vi "TPNT_PeriodicUpdate.vi"(4 "deflogsep":string="blank", 5 "UTC":bool, 6 "notifier":refnum<notifier>, 7 "mailserver":string="localhost", 9 "log":bool, 10 "logfile":path, 11 "queueIn":refnum<queue>) -> ()   [LabVIEW 2016]
uses:
  TPNT_CoreFunction.ctl
  TPNT_Refnum.ctl
panel:
  in  "sample now":bool
  in  "pause":bool
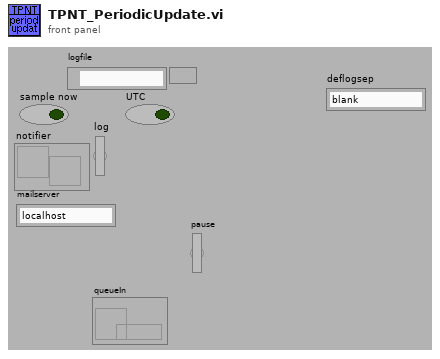
[diagram p1: front panel]
types:
  T1 = typedef "TPNT_Refnum.ctl" = refnum<vi>
  T2 = typedef "TPNT_CoreFunction.ctl" = enum16{"Reset", "Register", "Get Data", "Set Data", "Unregister", "Test", "Get Objects"}
  T3 = typedef "TPNT_TP.ctl" = cluster{"name":string, "type":string, "algor":string[], "update_rate":sgl, "Limits":T4, "Samples":T5, "next_update":u32, "Status":string, "monitor":bool, "error":bool, "Log":T6, "permissions":string, "ID":string}
  T4 = typedef "TPNT_Limits.ctl" = cluster{"Alarm Type":string, "Lower ":dbl, "Upper":dbl, "Nominal":dbl, "outrange":bool, "Check":bool, "latch":bool, "level":string}
  T5 = typedef "TPNT_Samples.ctl" = cluster{"samples":i32, "counter":i32, "Values":dbl[], "Current Value":string, "filter":string, "precision":u8}
  T6 = typedef "TPNT_Log.ctl" = cluster{"log":bool, "file":path, "type":string, "format":string, "updaterate":dbl, "nex_update":u32, "mode":string}
  T7 = typedef "TPNT_DeviceTPs.ctl" = cluster{"device":string, "devupdate":dbl, "next_update":u32, "devinterface":string, "TPs":T3[], "Alarms":bool, "monitor":bool, "log sep":string}
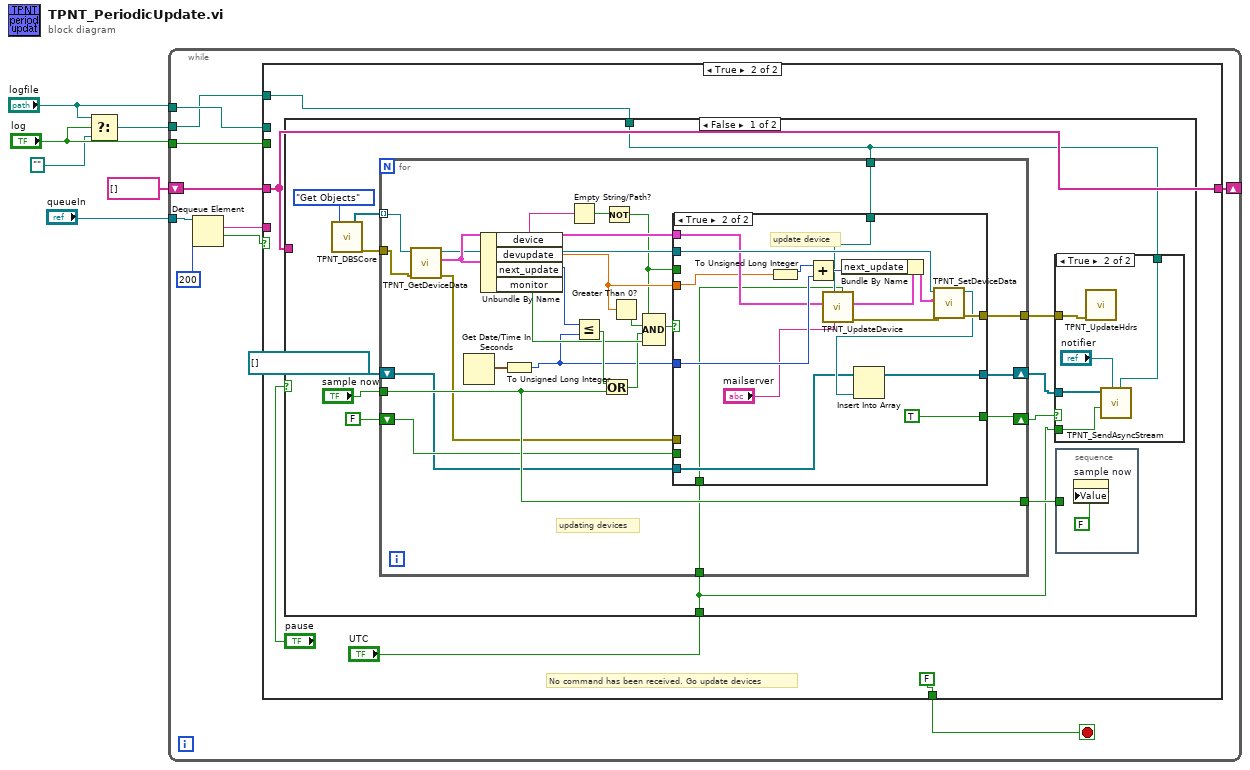
[diagram p0: block diagram]
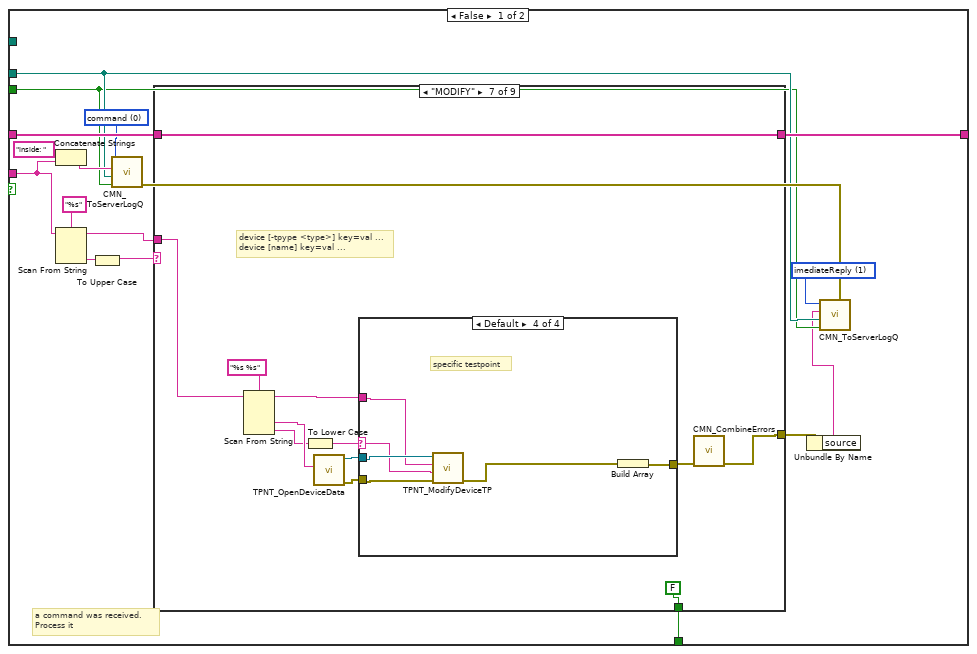
[diagram p2: hidden frame]
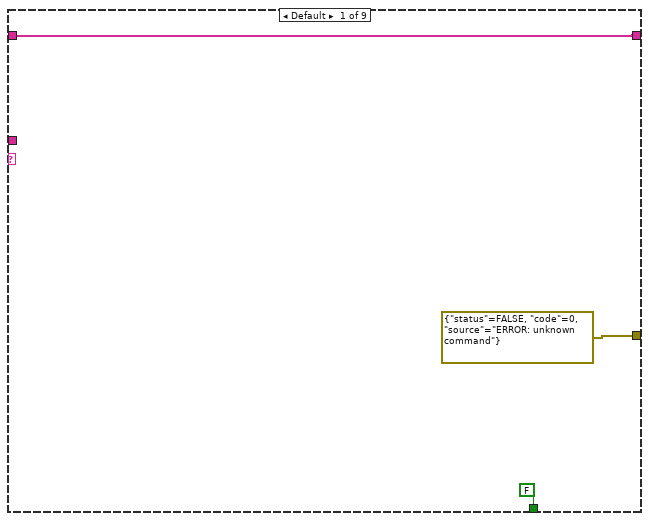
[diagram p3: hidden frame]
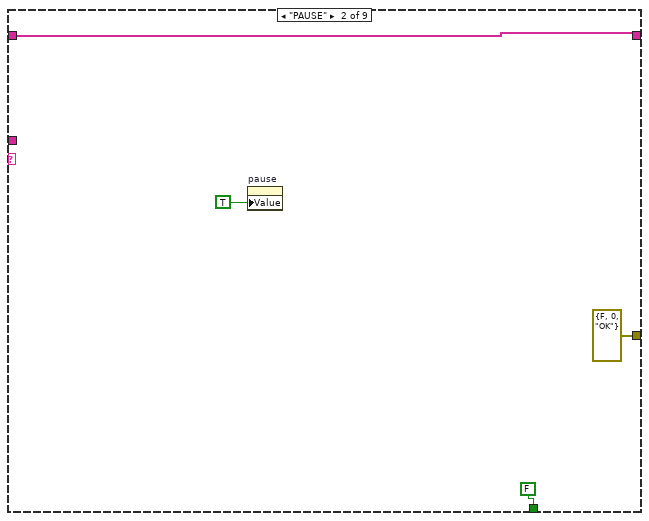
[diagram p4: hidden frame]
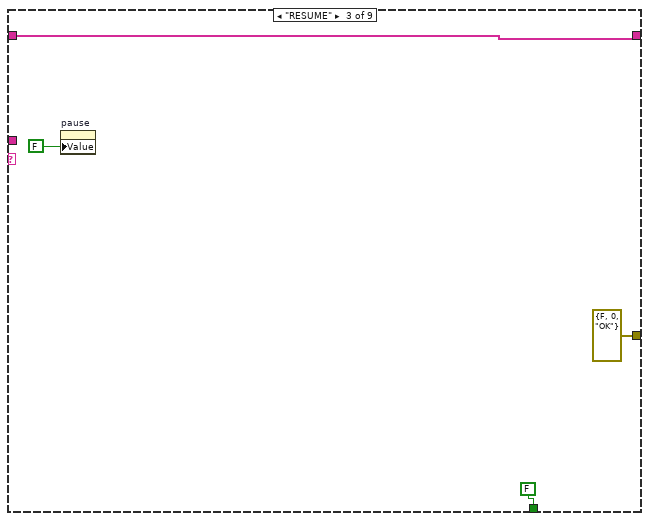
[diagram p5: hidden frame]
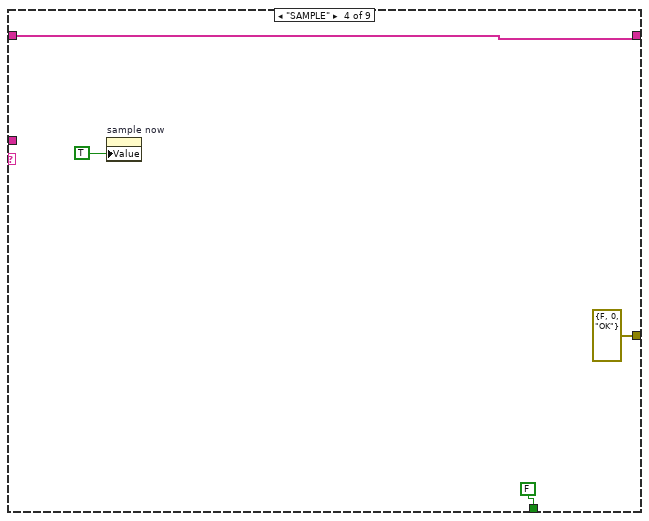
[diagram p6: hidden frame]
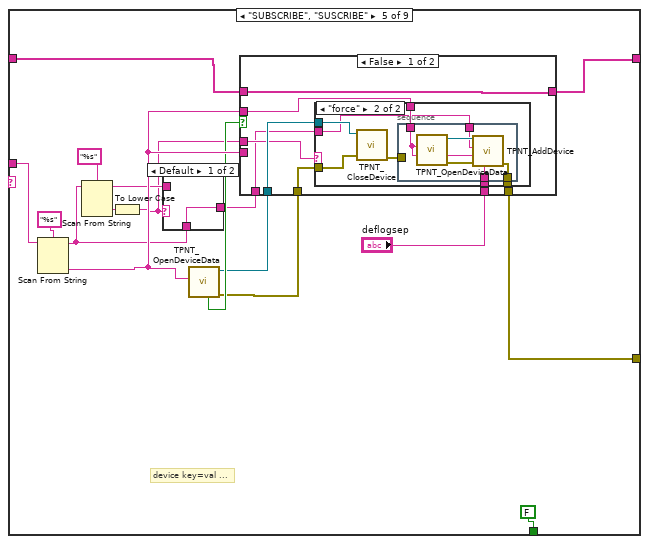
[diagram p7: hidden frame]
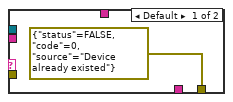
[diagram p9: hidden frame]
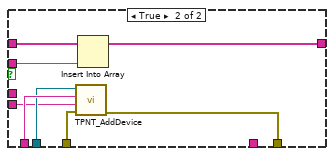
[diagram p10: hidden frame]
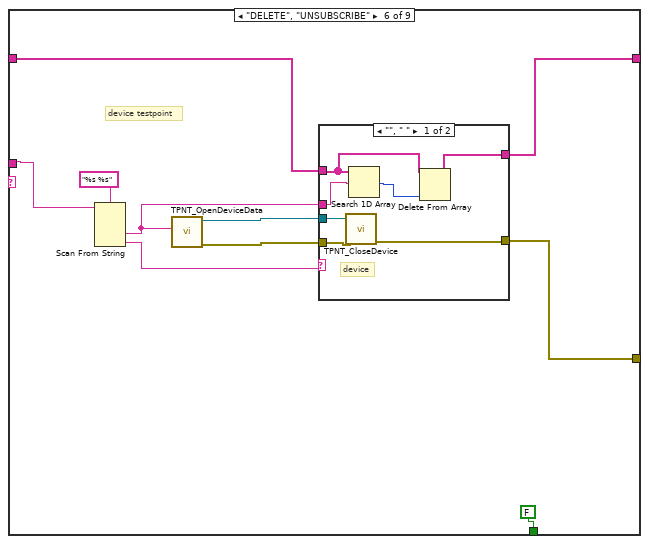
[diagram p11: hidden frame]
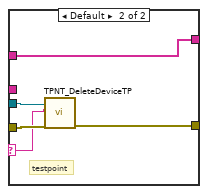
[diagram p12: hidden frame]
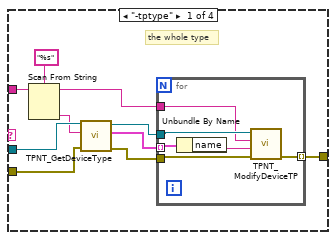
[diagram p13: hidden frame]
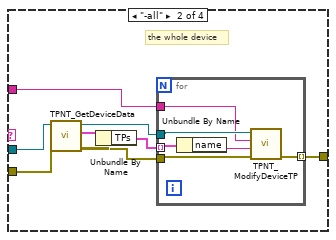
[diagram p14: hidden frame]
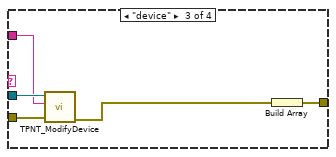
[diagram p15: hidden frame]
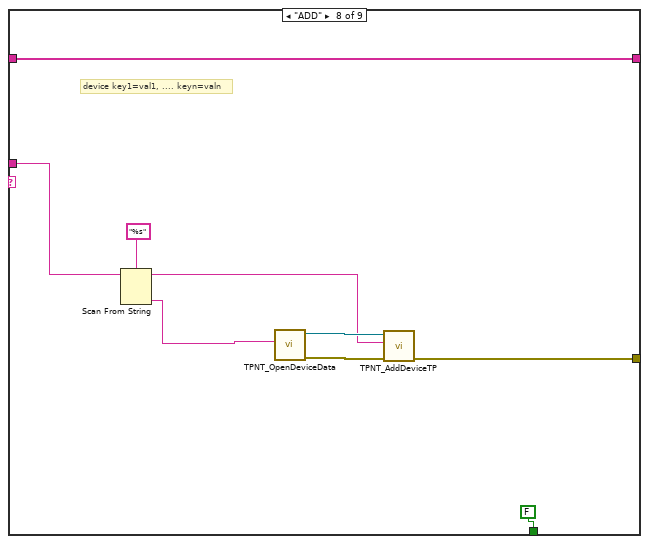
[diagram p16: hidden frame]
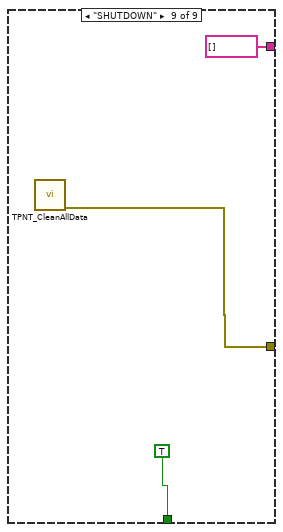
[diagram p17: hidden frame]
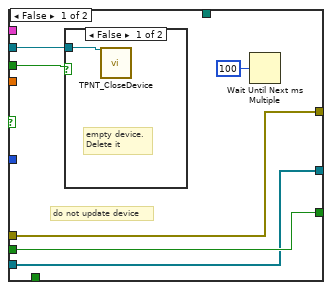
[diagram p19: hidden frame]
diagram:
  n1 = Select(t="logfile", s="log", f=path "") -> (s? t:f=w1:path)
  n2 = while {
    tunnel: "queueIn" -> [w16]
    shift-right: [w12] -> _
    shift-left: string[] [] -> [w10]
    tunnel: "log" -> [w9]
    tunnel: "logfile" -> [w8]
    tunnel: w1 -> [w7]
    stop <- w11 stop-if-true
    n3 = Dequeue Element(queue=w16, timeout in ms (-1)=200) -> (element=w13:string, timed out?=w14:bool)  [unwired: 1 in, 2 out]
    n4 = case shown="True" w14 {
      tunnel: w10 -> [w29 w188]
      tunnel: w13 -> [w24 _]
      tunnel: [w28 w188] -> w12
      tunnel: [w27 FALSE] -> w11
      tunnel: w9 -> [w20 _]
      tunnel: w8 -> [w21 _]
      tunnel: w7 -> [_ w186]
      frame False {
        w19 = u16 1 items=["command", "imediateReply", "Callback Reply", "Information"] ("type")
        w26 = u16 0 items=["command", "imediateReply", "Callback Reply", "Information"] ("type")
        # "a command was received.\nProcess it"
        n5 = Concatenate Strings("inside: " ("string"), w24) -> (w23:string)
        n6 = Scan From String(format string="%s", input string=w24) -> (remaining string=w30:string, output 1=w33:string)  [unwired: 2 in, 3 out]
        n7 = To Upper Case(1:w33) -> (0:w31:string)
        n8 = call "CMN_ToServerLogQ.vi"("Log"=w20, "file"=w21, "string"=w23, "type"=w26) -> ("error out"=w22:errorcluster)  [unwired: 2 in, 4 out]
        n9 = case shown="\"MODIFY\"" w31 {
          tunnel: w30 -> [_ _ _ _ w64 w101 w124 w177 _]
          tunnel: w29 -> [w35 w39 w43 w48 w63 w99 w122 w175 _]
          tunnel: [w35 w39 w43 w48 w62 w100 w122 w175 string[] []] -> w28
          tunnel: [FALSE FALSE FALSE FALSE FALSE FALSE FALSE FALSE TRUE] -> w27
          tunnel: [errorcluster {"status"=FALSE, "code"=0, "source"="ERROR: unknown command"} ("error out") errorcluster {"status"=FALSE, "code"=0, "source"="OK"} ("error out") errorcluster {"status"=FALSE, "code"=0, "source"="OK"} ("error out") errorcluster {"status"=FALSE, "code"=0, "source"="OK"} ("error out") w56 w98 w120 w173 w182] -> w18
          frame Default {
          }
          frame "PAUSE" {
            n10 = property on="pause" class="Bool (strict)"("Value"=TRUE ("pause")) -> ()  [unwired: 2 in, 2 out]
          }
          frame "RESUME" {
            n11 = property on="pause" class="Bool (strict)"("Value"=FALSE ("pause")) -> ()  [unwired: 2 in, 2 out]
          }
          frame "SAMPLE" {
            n12 = property on="sample now" class="Bool (strict)"("Value"=TRUE ("sample now")) -> ()  [unwired: 2 in, 2 out]
          }
          frame "SUBSCRIBE", "SUSCRIBE" {
            # "device key=val ..."
            n13 = Scan From String(format string="%s", input string=w64) -> (remaining string=w52:string, output 1=w60:string)  [unwired: 2 in, 3 out]
            n14 = Scan From String(format string="%s", input string=w52) -> (remaining string=w51:string, output 1=w54:string)  [unwired: 2 in, 3 out]
            n15 = To Lower Case(string=w54) -> (all lower case string=w50:string)
            n16 = case shown="Default" w50 {
              tunnel: w52 -> [w66 _]
              tunnel: [w66 w67] -> w53
              tunnel: w51 -> [_ w67]
              frame Default {
              }
              frame "force" {
              }
            }
            n17 = call "TPNT_OpenDeviceData.vi"("Name"=w60) -> ("error out"=w57:errorcluster, "Data Refnum out"=w58:T1, "Created New"=w59:bool)  [unwired: 1 in, 7 out]
            n18 = case shown="False" w59 {
              tunnel: w63 -> [w75 w97]
              tunnel: [w75 w96] -> w62
              tunnel: w60 -> [w70 w95]
              tunnel: w53 -> [w69 w94]
              tunnel: w58 -> [w74 w93]
              tunnel: w57 -> [w73 w92]
              tunnel: w60 -> [_ w91]
              tunnel: [w72 w90] -> w56
              tunnel: w50 -> [w71 _]
              tunnel: "deflogsep" -> [w68 _]
              frame False {
                n19 = case shown="\"force\"" w71 {
                  tunnel: w74 -> [_ w81]
                  tunnel: w73 -> [_ w83]
                  tunnel: [errorcluster {"status"=FALSE, "code"=0, "source"="Device already existed"} ("error out") w82] -> w72
                  tunnel: w70 -> [_ w80]
                  tunnel: w69 -> [_ w78]
                  tunnel: w68 -> [_ w77]
                  frame Default {
                  }
                  frame "force" {
                    n20 = call "TPNT_CloseDevice.vi"("error in (no error)"=w83, "Object Refnum In"=w81) -> ("error out"=w79:errorcluster)  [unwired: 9 out]
                    n21 = stacked-sequence {
                      tunnel: [w89] -> w82
                      tunnel: w80 -> [w86]
                      tunnel: w79 -> [_]
                      tunnel: w78 -> [w85]
                      tunnel: w77 -> [w84]
                      frame #0 {
                        n22 = call "TPNT_OpenDeviceData.vi"("Name"=w86) -> ("error out"=w88:errorcluster, "Data Refnum out"=w87:T1)  [unwired: 1 in, 8 out]
                        n23 = call "TPNT_AddDevice.vi"("deflogsep"=w84, "error in (no error)"=w88, "name"=w86, "arguments"=w85, "Object Refnum In"=w87) -> ("error out"=w89:errorcluster)  [unwired: 6 out]
                      }
                    }
                  }
                }
              }
              frame True {
                n24 = call "TPNT_AddDevice.vi"("error in (no error)"=w92, "name"=w91, "arguments"=w94, "Object Refnum In"=w93) -> ("error out"=w90:errorcluster)  [unwired: 1 in, 6 out]
                n25 = Insert Into Array(array=w97, new element=w95) -> (w96:string[])  [unwired: 1 in]
              }
            }
          }
          frame "DELETE", "UNSUBSCRIBE" {
            # "device testpoint"
            n26 = Scan From String(format string="%s %s", input string=w101) -> (output 1=w102:string, output 2=w103:string)  [unwired: 2 in, 5 out]
            n27 = call "TPNT_OpenDeviceData.vi"("Name"=w102) -> ("error out"=w104:errorcluster, "Data Refnum out"=w105:T1)  [unwired: 1 in, 8 out]
            n28 = case shown="\"\", \" \"" w103 {
              selector: w103 -> [_ w117]
              tunnel: w105 -> [w113 w119]
              tunnel: w104 -> [w114 w118]
              tunnel: w102 -> [w109 _]
              tunnel: w99 -> [w110 w116]
              tunnel: [w111 w116] -> w100
              tunnel: [w108 w115] -> w98
              frame "", " " {
                # "device"
                n29 = call "TPNT_CloseDevice.vi"("error in (no error)"=w114, "Object Refnum In"=w113) -> ("error out"=w108:errorcluster)  [unwired: 9 out]
                n30 = Search 1D Array(1D array=w110, element=w109) -> (index of element=w112:i32)  [unwired: 1 out]
                n31 = Delete From Array(array=w110, index=w112) -> (array with subset deleted=w111:string[])  [unwired: 1 in, 1 out]
              }
              frame Default {
                # "testpoint"
                n32 = call "TPNT_DeleteDeviceTP.vi"("error in (no error)"=w118, "TP name"=w117, "Object Refnum In"=w119) -> ("error out"=w115:errorcluster)  [unwired: 8 out]
              }
            }
          }
          frame "MODIFY" {
            # "device [-tpype <type>] key=val ...\ndevice [name] key=val ..."
            n33 = Scan From String(format string="%s %s", input string=w124) -> (remaining string=w127:string, output 1=w130:string, output 2=w126:string)  [unwired: 2 in, 4 out]
            n34 = To Lower Case(string=w126) -> (all lower case string=w125:string)
            n35 = call "TPNT_OpenDeviceData.vi"("Name"=w130) -> ("error out"=w128:errorcluster, "Data Refnum out"=w129:T1)  [unwired: 1 in, 8 out]
            n36 = case shown="Default" w125 {
              selector: w125 -> [_ _ _ w169]
              tunnel: w129 -> [w140 w154 w165 w172]
              tunnel: w128 -> [w141 w155 w166 w171]
              tunnel: w127 -> [w136 w151 w164 w170]
              tunnel: [w132 w148 w162 w167] -> w121
              frame "-tptype" {
                # "the whole type"
                n37 = Scan From String(format string="%s", input string=w136) -> (remaining string=w133:string, output 1=w134:string)  [unwired: 2 in, 3 out]
                n38 = call "TPNT_GetDeviceType.vi"("error in (no error)"=w141, "tptype"=w134, "Object Refnum In"=w140) -> ("error out"=w138:errorcluster, "Type"=w139:T3[], "Data Refnum out"=w137:T1)  [unwired: 6 out]
                n39 = for {
                  tunnel: w138 -> [w146]
                  tunnel: w137 -> [w145]
                  tunnel: w139 -> [w147] mode=indexing
                  tunnel: w133 -> [w143]
                  tunnel: [w142] -> w132 mode=indexing
                  n40 = Unbundle By Name(w147) -> ("name"=w144:string)
                  n41 = call "TPNT_ModifyDeviceTP.vi"("error in (no error)"=w146, "name"=w144, "arguments"=w143, "Object Refnum In"=w145) -> ("error out"=w142:errorcluster)  [unwired: 7 out]
                }
              }
              frame "-all" {
                # "the whole device"
                n42 = call "TPNT_GetDeviceData.vi"("error in (no error)"=w155, "Object Refnum In"=w154) -> ("error out"=w153:errorcluster, "Object Data Out"=w150:T7, "Data Refnum out"=w152:T1)  [unwired: 7 out]
                n43 = Unbundle By Name(w150) -> ("TPs"=w149:T3[])
                n44 = for {
                  tunnel: w153 -> [w160]
                  tunnel: w152 -> [w159]
                  tunnel: w149 -> [w161] mode=indexing
                  tunnel: w151 -> [w157]
                  tunnel: [w156] -> w148 mode=indexing
                  n45 = Unbundle By Name(w161) -> ("name"=w158:string)
                  n46 = call "TPNT_ModifyDeviceTP.vi"("error in (no error)"=w160, "name"=w158, "arguments"=w157, "Object Refnum In"=w159) -> ("error out"=w156:errorcluster)  [unwired: 7 out]
                }
              }
              frame "device" {
                n47 = call "TPNT_ModifyDevice.vi"("error in (no error)"=w166, "arguments"=w164, "Object Refnum In"=w165) -> ("error out"=w163:errorcluster)  [unwired: 8 out]
                n48 = Build Array(w163) -> (w162:errorcluster[])
              }
              frame Default {
                # "specific testpoint"
                n49 = call "TPNT_ModifyDeviceTP.vi"("error in (no error)"=w171, "name"=w169, "arguments"=w170, "Object Refnum In"=w172) -> ("error out"=w168:errorcluster)  [unwired: 7 out]
                n50 = Build Array(w168) -> (w167:errorcluster[])
              }
            }
            n51 = call "CMN_CombineErrors.vi"("Errors"=w121) -> ("error out"=w120:errorcluster)  [unwired: 10 out]
          }
          frame "ADD" {
            # "device key1=val1, .... keyn=valn"
            n52 = Scan From String(format string="%s", input string=w177) -> (remaining string=w174:string, output 1=w178:string)  [unwired: 2 in, 3 out]
            n53 = call "TPNT_OpenDeviceData.vi"("Name"=w178) -> ("error out"=w180:errorcluster, "Data Refnum out"=w179:T1)  [unwired: 1 in, 8 out]
            n54 = call "TPNT_AddDeviceTP.vi"("error in (no error)"=w180, "arguments"=w174, "Object Refnum In"=w179) -> ("error out"=w173:errorcluster)  [unwired: 8 out]
          }
          frame "SHUTDOWN" {
            n55 = call "TPNT_CleanAllData.vi"() -> ("error out"=w182:errorcluster)  [unwired: 1 in, 10 out]
          }
        }
        n56 = Unbundle By Name(w18) -> ("source"=w17:string)
        n57 = call "CMN_ToServerLogQ.vi"("error in (no error)"=w22, "Log"=w20, "file"=w21, "string"=w17, "type"=w19) -> ()  [unwired: 1 in, 5 out]
      }
      frame True {
        # "No command has been received. Go update devices"
        n58 = case shown="False" "pause" {
          tunnel: w188 -> [_ _]
          tunnel: w186 -> [w190 _]
          tunnel: "UTC" -> [w191 _]
          frame False {
            n59 = call "TPNT_DBSCore.vi"("Function (Get Data)"=TPNT_CoreFunction."Get Objects") -> ("Objects"=w201:T1[], "error out"=w200:errorcluster)  [unwired: 4 in, 13 out]
            n60 = for {
              tunnel: w201 -> [w225] mode=indexing
              tunnel: w200 -> [w224]
              tunnel: w190 -> [w219]
              tunnel: "sample now" -> [w217]
              tunnel: [w217] -> w197
              tunnel: [w216] -> w196
              shift-right: [w214] -> w194
              shift-left: FALSE -> [w213]
              shift-right: [w212] -> w192
              shift-left: T1[] [] -> [w211]
              tunnel: w191 -> [w208]
              # "updating devices"
              n61 = call "TPNT_GetDeviceData.vi"("error in (no error)"=w224, "Object Refnum In"=w225) -> ("error out"=w215:errorcluster, "Object Data Out"=w228:T7, "Data Refnum out"=w227:T1)  [unwired: 7 out]
              n62 = Get Date/Time In Seconds() -> (seconds since 1Jan1904=w209:timestamp)
              n63 = Unbundle By Name(w228) -> ("device"=w222:string, "devupdate"=w226:dbl, "next_update"=w230:u32, "monitor"=w223:bool)
              n64 = To Unsigned Long Integer(number=w209) -> (unsigned 32bit integer=w210:u32)
              n65 = Empty String/Path?(string/path=w222) -> (empty?=w221:bool)
              n66 = Less Or Equal?(x=w230, y=w210) -> (x <= y?=w229:bool)
              n67 = Or(x=w229, y=w217) -> (x .or. y?=w218:bool)
              n68 = Not(x=w221) -> (.not. x?=w220:bool)
              n69 = Greater Than 0?(x=w226) -> (x > 0?=w232:bool)
              n70 = Compound Arithmetic op=AND(w220, w232, w218, w223) -> (w231:bool)
              n71 = case shown="True" w231 {
                tunnel: w210 -> [_ w252]
                tunnel: w228 -> [_ w246]
                tunnel: w227 -> [w236 w256]
                tunnel: w226 -> [_ w242]
                tunnel: w220 -> [w237 _]
                tunnel: w219 -> [_ w249]
                tunnel: [w235 w248] -> w216
                tunnel: w215 -> [w235 _]
                tunnel: [w234 TRUE] -> w214
                tunnel: w213 -> [w234 _]
                tunnel: [w233 w245] -> w212
                tunnel: w211 -> [w233 w243]
                tunnel: w208 -> [_ w240]
                frame False {
                  # "do not update device"
                  n72 = case shown="False" w237 {
                    tunnel: w236 -> [w239 _]
                    frame False {
                      # "empty device.\nDelete it"
                      n73 = call "TPNT_CloseDevice.vi"("Object Refnum In"=w239) -> ()  [unwired: 1 in, 10 out]
                    }
                    frame True {
                    }
                  }
                  n74 = Wait Until Next ms Multiple(millisecond multiple=u32 100) -> ()  [unwired: 1 out]
                }
                frame True {
                  # "update device"
                  n75 = To Unsigned Long Integer(number=w242) -> (unsigned 32bit integer=w253:u32)
                  n76 = Add(x=w253, y=w252) -> (x+y=w251:u32)
                  n77 = call "TPNT_UpdateDevice.vi"("UTC"=w240, "mailserver"="mailserver", "tpnt_logfile"=w249, "Device In"=w246) -> ("error out"=w255:errorcluster, "Device IOut"=w254:T7)  [unwired: 1 in, 5 out]
                  n78 = Bundle By Name(cluster=w254, "next_update"=w251) -> (w250:T7)
                  n79 = call "TPNT_SetDeviceData.vi"("error in (no error)"=w255, "Object Data In"=w250, "Object Refnum In"=w256) -> ("error out"=w248:errorcluster, "Data Refnum out"=w244:T1)  [unwired: 7 out]
                  n80 = Insert Into Array(array=w243, new element=w244) -> (w245:T1[])  [unwired: 1 in]
                }
              }
            }
            n81 = case shown="True" w194 {
              tunnel: w196 -> [_ w206]
              tunnel: w192 -> [_ w205]
              tunnel: w191 -> [_ w203]
              tunnel: w190 -> [_ w202]
              frame False {
              }
              frame True {
                n82 = call "TPNT_UpdateHdrs.vi"("error in (no error)"=w206) -> ()  [unwired: 11 out]
                n83 = call "TPNT_SendAsyncStream.vi"("logfile"=w202, "notifier"="notifier", "UTC"=w203, "Objects"=w205) -> ()  [unwired: 8 out]
              }
            }
            n84 = stacked-sequence {
              tunnel: w197 -> [_]
              frame #0 {
                n85 = property on="sample now" class="Bool (strict)"("Value"=FALSE ("sample now")) -> ()  [unwired: 2 in, 2 out]
              }
            }
          }
          frame True {
            # "we are paused"
          }
        }
      }
    }
  }
